vi "RunOperation.vi"(10 "Inputs":string[](array[string]), 11 "Test in":refnum<class "Test.lvclass">) -> (1 "Output/Failure":string, 2 "CLI Process Return Code":i32, 3 "Test out":refnum<class "Test.lvclass">)   [LabVIEW 2017, in "Test.lvclass"]
uses:
  Test.lvclass
  Test.lvclass/Test.ctl
  <vilib>/PNR/Caraya JUnit for Azure Pipelines/JUnit for Azure Pipelines/JUnit for Azure Pipelines.lvclass
  C:/Program Files (x86)/National Instruments/LabVIEW 2017/vi.lib/addons/_JKI Toolkits/Caraya/classes/Test Report/Test Report.lvclass
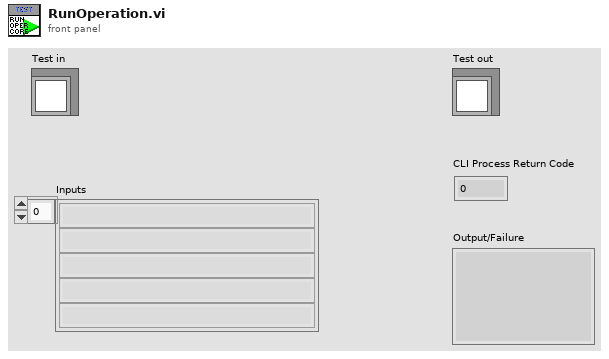
[diagram p1: front panel]
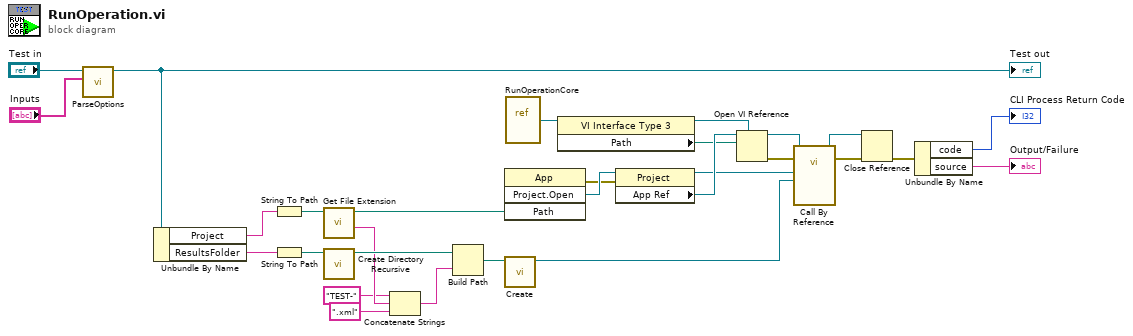
[diagram p0: block diagram]
diagram:
  n1 = call "ParseOptions.vi"("Options"="Inputs", "Test in"="Test in") -> ("Test out"=w25:refnum<class "Test.lvclass">)  [unwired: 8 in, 1 out]
  "Test out" <- w25
  n2 = Unbundle By Name(w25) -> ("Project"=w24:string, "ResultsFolder"=w12:string)
  n3 = String To Path(string=w24) -> (path=w8:path)
  n4 = String To Path(string=w12) -> (path=w10:path)
  n5 = call <vilib>:"Get File Extension.vi"("file"=w8) -> ("filename without extension"=w7:string, "dup file"=w3:path)  [unwired: 6 in, 3 out]
  n6 = call <vilib>:"Create Directory Recursive.vi"("directory"=w10) -> ("directory copy"=w9:path)  [unwired: 4 in, 2 out]
  n7 = Concatenate Strings("TEST-" ("string"), w7, ".xml" ("string")) -> (w4:string)
  n8 = Build Path(base path=w9, name or relative path=w4) -> (appended path=w2:path)
  n9 = invoke class="App" method="Project.Open"("Path"=w3) -> (error out=w13:errorcluster, "Project:Open"=w15:refnum<vi>)  [unwired: 3 in, 2 out]
  n10 = call <vilib>:"Create.vi"("Path"=w2) -> ("JUnit for Azure Pipelines"=w1:refnum<class "JUnit for Azure Pipelines.lvclass">)  [unwired: 9 in, 1 out]
  n11 = vi-ref "RunOperationCore.vi"() -> (w20:refnum<vi>)
  n12 = property class="VI Interface Type 3"(reference=w20) -> (reference out=w18:refnum<vi>, "Path"=w19:path)  [unwired: 1 in, 1 out]
  n13 = property class="Project"(reference=w15, error in=w13) -> (reference out=w14:refnum<vi>, "App Ref"=w21:refnum<vi>)  [unwired: 1 out]
  n14 = Open VI Reference(type specifier VI Refnum (for type only)=w18, application reference (local)=w21, vi path=w19) -> (vi reference=w16:refnum<vi>, error out=w22:errorcluster)  [unwired: 3 in]
  n15 = call-by-ref "?"(reference=w16, error in=w22, "Test Report"=w1, "Project"=w14) -> (reference out=w11:refnum<vi>, error out=w17:errorcluster)  [unwired: 9 in, 1 out]
  n16 = Close Reference(reference=w11, error in (no error)=w17) -> (error out=w23:errorcluster)
  n17 = Unbundle By Name(w23) -> ("code"=→"CLI Process Return Code":i32, "source"=→"Output/Failure":string)
